vi "Configure Digital Input Noise Multiplex.vi"(8 "error in (no error)":errorcluster, 10 "Output Multiplex (0: Carrier+Noise)":i32(ring) items=["Carrier+Noise", "Carrier", "Noise"], 11 "VISA resource name":refnum<visa-resource-name>) -> (0 "error out":errorcluster, 3 "VISA resource name out":refnum<visa-resource-name>)   [LabVIEW 2018, in "Agilent PSG MXG Series.lvlib"]
doc: "Configures the diagnostic control of additive noise.\n\n<b>Note:</b>\nIt is applicable for N5172B/82B with <b>Option 004</b> only."
uses:
  Agilent PSG MXG Series.lvlib
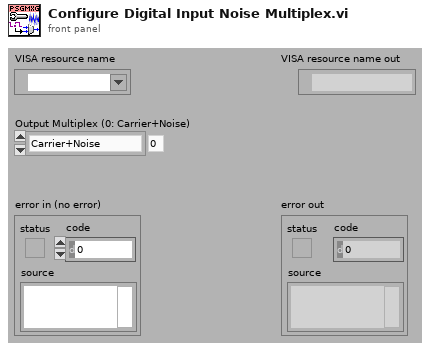
[diagram p1: front panel]
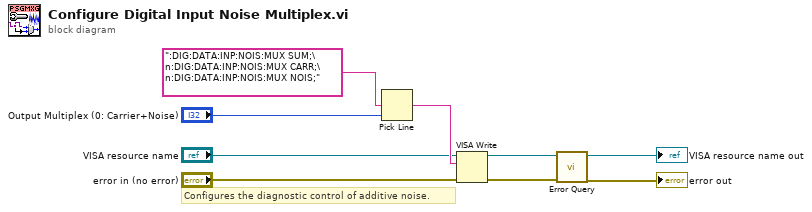
[diagram p0: block diagram]
diagram:
  # "Configures the diagnostic control of additive noise."
  n1 = Pick Line(multi-line string=":DIG:DATA:INP:NOIS:MUX SUM;\n:DIG:DATA:INP:NOIS:MUX CARR;\n:DIG:DATA:INP:NOIS:MUX NOIS;", line index="Output Multiplex (0: Carrier+Noise)") -> (output string=w7:string)  [unwired: 1 in]
  n2 = VISA Write(VISA resource name="VISA resource name", write buffer=w7, error in (no error)="error in (no error)") -> (VISA resource name out=w4:refnum<visa-resource-name>, error out=w3:errorcluster)  [unwired: 1 out]
  n3 = call "Error Query.vi"("error in (no error)"=w3, "VISA resource name"=w4) -> ("error out"=→"error out":errorcluster, "VISA resource name out"=→"VISA resource name out":refnum<visa-resource-name>)  [unwired: 6 in, 2 out]
